vi "Save Image.vi"(8 "error in (no error)":errorcluster, 11 "CCD in":refnum<class "CCD.lvclass">) -> (0 "error out":errorcluster, 3 "CCD out":refnum<class "CCD.lvclass">)   [LabVIEW 2018, in "CCD.lvclass"]
uses:
  CCD.lvclass
  <userlib>/gfitsio/cfitsio-bitpix.ctl
  CCD.lvclass/CCD.ctl
  <userlib>/gfitsio/gfitsio-write-image-subset-i16-3d.vi
  <userlib>/gfitsio/gfitsio.lvlib
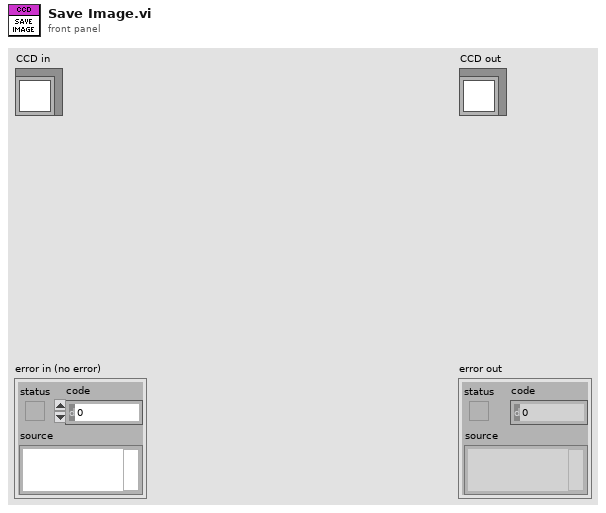
[diagram p1: front panel]
types:
  T1 = enum16{"open", "open or create", "create or replace", "create", "open (read only)"}
  T2 = enum16{"open", "open or create", "create", "create or replace"}
  T3 = typedef "gfitsio.lvlib/cfitsio-bitpix.ctl" = i32
  T4 = typedef "gfitsio.lvlib/gfitsio-refnum.ctl" = refnum<k1>
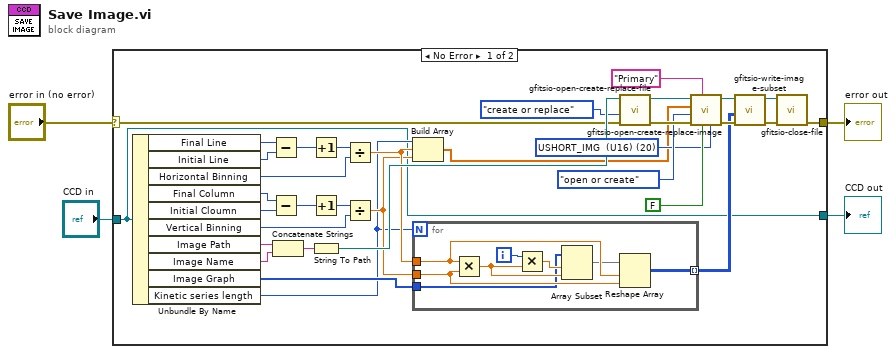
[diagram p0: block diagram]
diagram:
  n1 = case shown="No Error" "error in (no error)" {
    selector: "error in (no error)" -> [w8 w48]
    tunnel: [w38 w48] -> w1
    tunnel: [w9 w47] -> w2
    tunnel: "CCD in" -> [w9 w47]
    frame No Error {
      w33 = T3 20 items=["<invalid type>"=0, "BYTE_IMG  (U8)"=8, "SHORT_IMG  (I16)"=16, "USHORT_IMG  (U16)"=20, "LONG_IMG  (I32)"=32, "ULONG_IMG  (U32)"=40, "FLOAT_IMG  (SGL)"=-32, "DOUBLE_IMG  (DBL)"=-64] ("image data type")
      n2 = Unbundle By Name(w9) -> ("Final Line"=w24:u16, "Initial Line"=w25:u16, "Horizontal Binning"=w26:u16, "Final Column"=w27:u16, "Initial Cloumn"=w28:u16, "Vertical Binning"=w29:u16, "Image Path"=w7:string, "Image Name"=w6:string, "Image Graph"=w11:u16[], "Kinetic series length"=w10:u32)
      n3 = Subtract(x=w24, y=w25) -> (x-y=w20:u16)
      n4 = Subtract(x=w27, y=w28) -> (x-y=w21:u16)
      n5 = Concatenate Strings(w7, w6) -> (w5:string)
      n6 = Increment(x=w20) -> (x+1=w22:u16)
      n7 = Increment(x=w21) -> (x+1=w23:u16)
      n8 = String To Path(string=w5) -> (path=w32:path)
      n9 = Divide(x=w22, y=w26) -> (x/y=w19:dbl)
      n10 = Divide(x=w23, y=w29) -> (x/y=w18:dbl)
      n11 = Build Array(w10, w19, w18) -> (w17:dbl[])
      n12 = for {
        N: w10 -> [_]
        tunnel: w11 -> [w41]
        tunnel: w19 -> [w46]
        tunnel: w18 -> [w45]
        tunnel: [w39] -> w12 mode=indexing
        i -> [w44]
        n13 = Multiply(x=w46, y=w45) -> (x*y=w43:dbl)
        n14 = Multiply(x=w44, y=w43) -> (x*y=w42:dbl)
        n15 = Array Subset(array=w41, index=w42, length=w43) -> (w40:u16[])
        n16 = Reshape Array(w40, w46, w45) -> (w39:u16[][])
      }
      n17 = call <userlib>:"gfitsio-open-create-replace-file.vi"("error in (no error)"=w8, "function (open)"=T1."create or replace", "file path (dialog if empty)"=w32) -> ("error out"=w37:errorcluster, "gfits refnum"=w36:T4)  [unwired: 6 in, 1 out]
      n18 = call <userlib>:"gfitsio-open-create-replace-image.vi"("image data type"=w33, "advisory dialog? (display:T)"=FALSE, "hdu name (dialog if empty)"="Primary" ("prompt"), "error in (no error)"=w37, "function (open or create)"=T2."open or create", "naxes"=w17, "gfits refnum"=w36) -> ("error out"=w13:errorcluster, "dup gfits refnum"=w14:T4)  [unwired: 2 in, 1 out]
      n19 = call-poly <userlib>:"gfitsio-write-image-subset.vi"("error in (no error)"=w13, "data"=w12, "gfits refnum"=w14) -> ("error out"=w16:errorcluster, "dup gfits refnum"=w15:T4)  [unwired: 7 in]
      n20 = call <userlib>:"gfitsio-close-file.vi"("error in (no error)"=w16, "gfits refnum"=w15) -> ("error out"=w38:errorcluster)  [unwired: 8 in, 1 out]
    }
    frame Error {
    }
  }
  "error out" <- w1
  "CCD out" <- w2
